vi "Get File Size.vi"(8 "error in (no error)":errorcluster, 11 "Text File in":refnum<class "Text File.lvclass">) -> (0 "error out":errorcluster, 2 "size (in bytes)":i64, 3 "Text File out":refnum<class "Text File.lvclass">)   [LabVIEW 2019, in "Text File.lvclass"]
uses:
  <vilib>/gpm_packages/@cs/event-logger/Source/Text File Sink/Text File/Text File.lvclass
  <vilib>/gpm_packages/@cs/event-logger/Source/Text File Sink/Text File/Text File.lvclass/Text File.ctl
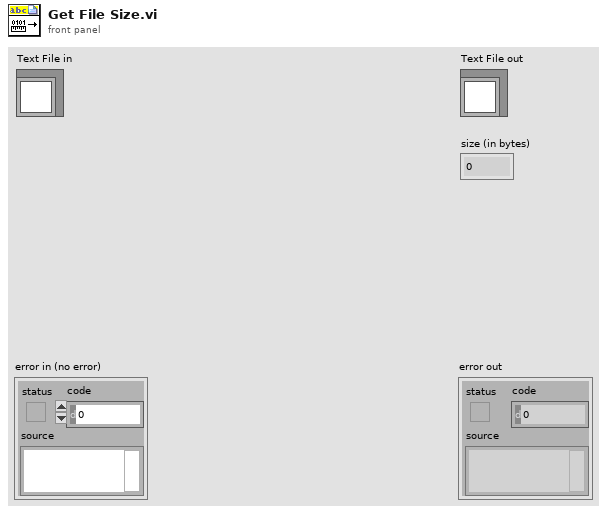
[diagram p1: front panel]
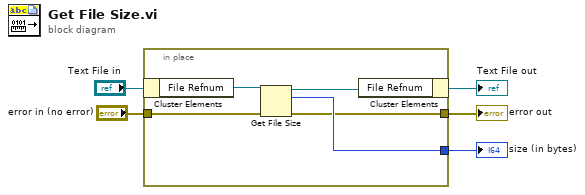
[diagram p0: block diagram]
diagram:
  n1 = in-place {
    in-place-border: [w8] -> w3
    in-place-border: "error in (no error)" -> [w7]
    in-place-border: [w6] -> w1
    n2 = in-place-cluster #1("Text File in") -> ("File Refnum"=w10:refnum<file>)
    n3 = Get File Size(file=w10, error in=w7) -> (refnum out=w9:refnum<file>, size (in bytes)=w8:i64, 0:w6:errorcluster)
    n4 = in-place-cluster #1("File Refnum"=w9) -> (→"Text File out":refnum<class "Text File.lvclass">)
  }
  "error out" <- w1
  "size (in bytes)" <- w3
